vi "ConfClose.vi"(8 "error in":errorcluster, 10 "Write?":bool=TRUE, 11 "StructIn":T1) -> (0 "error out":errorcluster, 3 "StructOut":T1)   [LabVIEW 2021, in "LibDan.lvlib"]
uses:
  LibDan.lvlib
  TerminalDef.ctl
  <vilib>/Utility/config.llb/Config Data RefNum.ctl
  <vilib>/Utility/config.llb/NI_LVConfig.lvlib
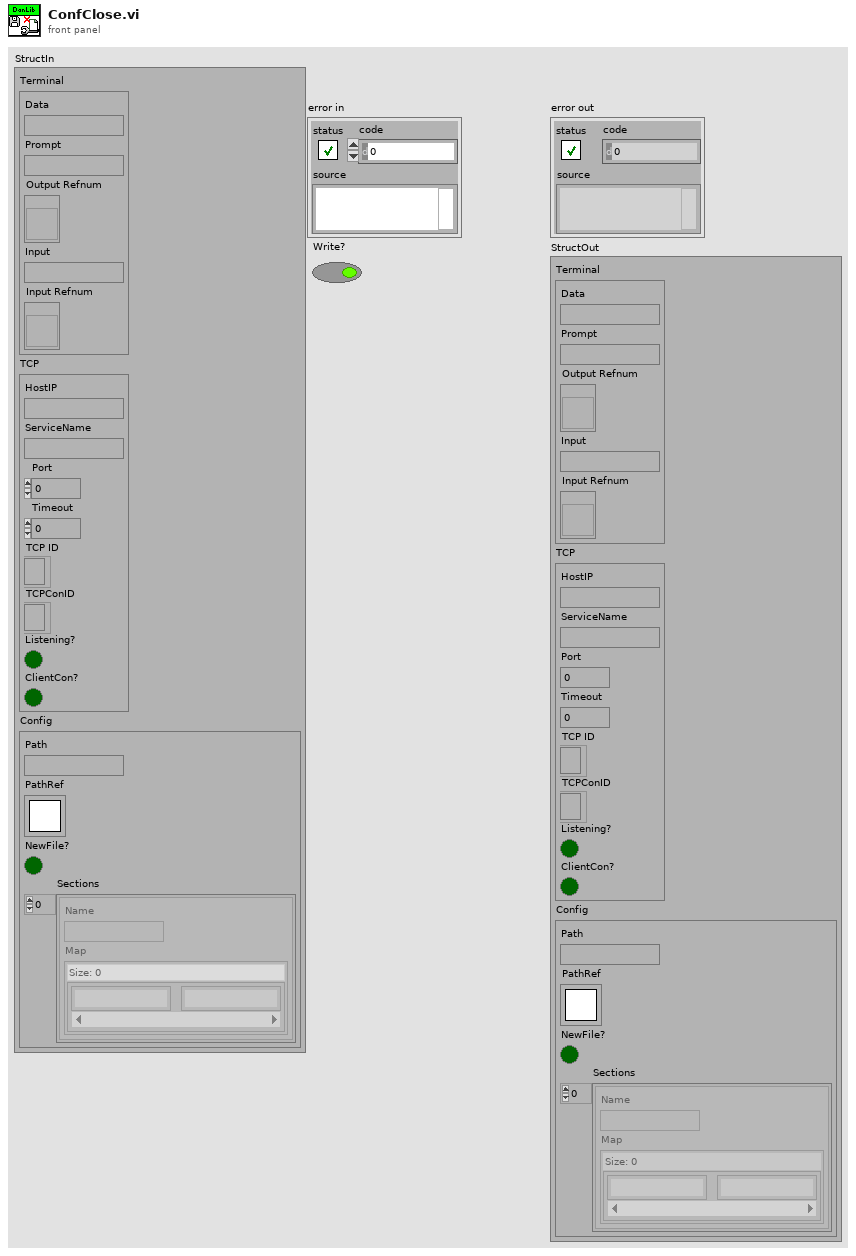
[diagram p1: front panel]
types:
  T1 = typedef "LibDan.lvlib/TerminalDef.ctl" = cluster{"Terminal":cluster{"Data":string, "Prompt":string, "Output Refnum":refnum<vi>, "Input":string, "Input Refnum":refnum<vi>}, "TCP":cluster{"HostIP":string, "ServiceName":string, "Port":u16, "Timeout":i32, "TCP ID":refnum<k5>, "TCPConID":refnum<k5>, "Listening?":bool, "ClientCon?":bool}, "Config":cluster{"Path":path, "PathRef":T2, "NewFile?":bool, "Sections":cluster{"Name":string, "Map":map{string, string}}[]}}
  T2 = typedef "NI_LVConfig.lvlib/Config Data RefNum.ctl" = refnum<k1>
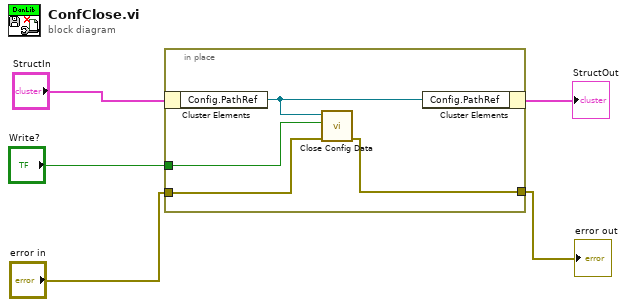
[diagram p0: block diagram]
diagram:
  n1 = in-place {
    in-place-border: "error in" -> [w9]
    in-place-border: "Write?" -> [w7]
    in-place-border: [w8] -> w2
    n2 = in-place-cluster #1("StructIn") -> ("Config.PathRef"=w6:T2)
    n3 = call <vilib>:"Close Config Data.vi"("error in (no error)"=w9, "write file if changed (T)"=w7, "refnum"=w6) -> ("error out"=w8:errorcluster)  [unwired: 7 in, 1 out]
    n4 = in-place-cluster #1("Config.PathRef"=w6) -> (→"StructOut":T1)
  }
  "error out" <- w2
